vi "Handle Last Ack Core.vi"(4 "error in (no error)":errorcluster, 6 "Last Ack":refnum<class "Last Ack.lvclass">, 7 "Jobber Proxy in":refnum<class "Jobber Proxy.lvclass">) -> (0 "error out":errorcluster, 3 "Jobber Proxy out":refnum<class "Jobber Proxy.lvclass">)   [LabVIEW 2014, in "Jobber Proxy.lvlib" / "Jobber Proxy.lvclass"]
doc: "(<B>Filename</B>: Actor Framework.lvlib:Actor.lvclass:Handle Last Ack Core.vi)\n\nDefines how the caller actor responds to the Last Ack message from a nested actor. The Last Ack message is the final message a nested actor sends to its caller before it shuts down. The message contains information about the final state of the nested actor.\n\nBy default, this method does nothing except return any error the nested actor sent. A descendant class may override this method to define behavior."
uses:
  Jobber Proxy.lvclass
  <vilib>/ActorFramework/LastAck/Last Ack.lvclass
  Jobber/Jobber/Jobber.lvclass
  <vilib>/ActorFramework/LastAck/Last Ack.lvclass/Last Ack.ctl
  Jobber/Jobber/Jobber.lvclass/Jobber.ctl
  Jobber Proxy.lvclass/Jobber Proxy.ctl
  <vilib>/ActorFramework/Actor/Actor.lvclass
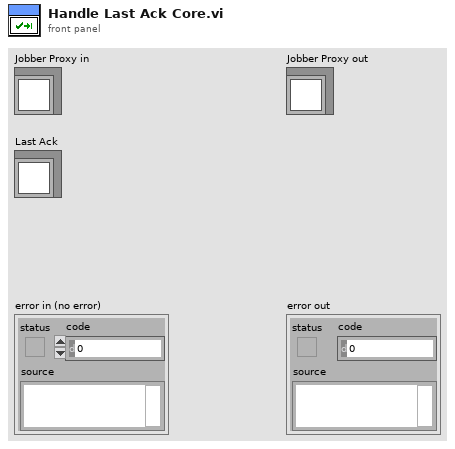
[diagram p1: front panel]
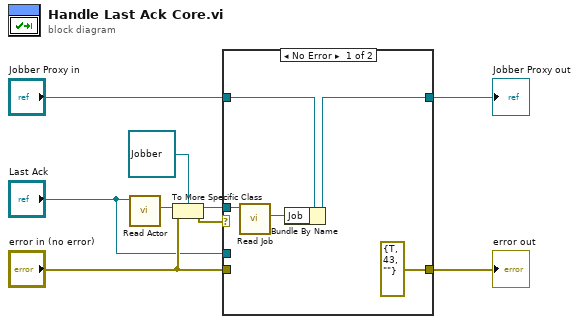
[diagram p0: block diagram]
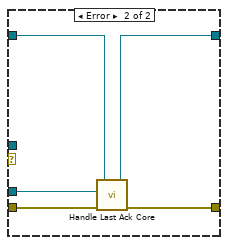
[diagram p2: hidden frame]
diagram:
  n1 = call <vilib>:"Read Actor.vi"("Last Ack"="Last Ack") -> ("Actor"=w8:refnum<class "Actor.lvclass">)  [unwired: 10 in]
  n2 = To More Specific Class(target class=refnum<class "Jobber.lvclass"> refnum ("Jobber in"), reference=w8, error in="error in (no error)") -> (specific class reference=w4:refnum<class "Jobber.lvclass">, error out=w3:errorcluster)
  n3 = case shown="No Error" w3 {
    tunnel: "Jobber Proxy in" -> [w12 w17]
    tunnel: [w11 w16] -> w5
    tunnel: [errorcluster {"status"=TRUE, "code"=43, "source"=""} ("error in") w18] -> w6
    tunnel: w4 -> [w13 _]
    tunnel: "error in (no error)" -> [_ w19]
    tunnel: "Last Ack" -> [_ w15]
    frame No Error {
      n4 = call "Read Job.vi"("Jobber in"=w13) -> ("Job.lvclass"=w14:refnum<class "Job.lvclass">)  [unwired: 10 in]
      n5 = Bundle By Name(cluster=w12, "Job"=w14) -> (w11:refnum<class "Jobber Proxy.lvclass">)
    }
    frame Error {
      n6 = call-parent "Handle Last Ack Core.vi"("error in (no error)"=w19, "Last Ack"=w15, "Actor in"=w17) -> ("error out"=w18:errorcluster, "Actor out"=w16:refnum<class "Jobber Proxy.lvclass">)  [unwired: 3 in]
    }
  }
  "Jobber Proxy out" <- w5
  "error out" <- w6
